vi "Create Output Channels.vi"(8 "error in (no error)":errorcluster, 11 "DAQmx Lockin Digitizer Driver in":refnum<class "DAQmx Lockin Digitizer Driver.lvclass">) -> (0 "error out":errorcluster, 3 "DAQmx Lockin Digitizer Driver out":refnum<class "DAQmx Lockin Digitizer Driver.lvclass">)   [LabVIEW 2021, in "DAQmx Lockin Digitizer Driver.lvclass"]
uses:
  DAQmx Lockin Digitizer Driver.lvclass
  C:/GitHub/NHMFL_Core/Libraries/Instruments/Pulse Driver/Lockin Digitizer Driver/Lockin Digitizer Driver.lvclass
  C:/GitHub/NHMFL_Core/Libraries/NI-DAQ/DAQmx Digitizer/DAQmx Digitizer.lvclass
  C:/GitHub/NHMFL_Core/Libraries/Instruments/Pulse Driver/Pulse Driver.lvclass
  DAQmx Digitizer/DAQmx Digitizer.lvclass/DAQmx Digitizer.ctl
  <vilib>/DAQmx/write.llb/DAQmx Write (Analog 2D DBL NChan NSamp).vi
  DAQmx Digitizer/Read DAQmx Device Name.vi
  <vilib>/DAQmx/create/channels.llb/DAQmx Create Channel (AO-Voltage-Basic).vi
  <vilib>/DAQmx/configure/timing.llb/DAQmx Timing (Sample Clock).vi
  <vilib>/DAQmx/miscellaneous.llb/DAQmx Fill In Error Info.vi
  DAQmx Lockin Digitizer Driver.lvclass/DAQmx Lockin Digitizer Driver.ctl
  <vilib>/Analysis/NI_AALBase.lvlib
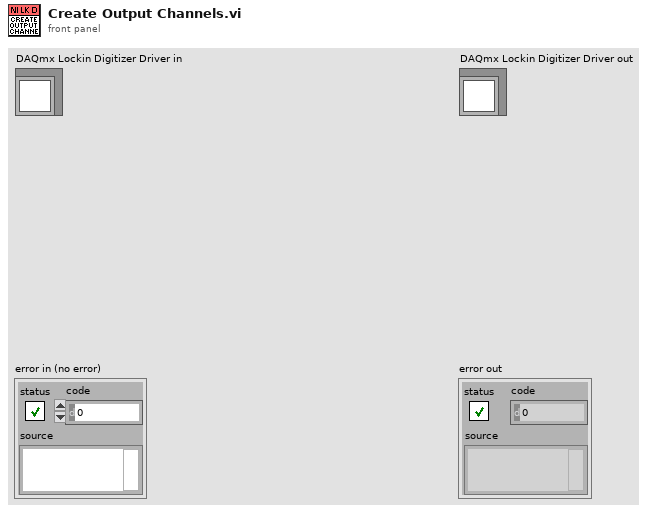
[diagram p1: front panel]
types:
  T1 = typedef "Lockin Digitizer Configuration.ctl" = cluster{"Post-trigger delay":dbl, "Post-trigger duration":dbl, "Rate":dbl, "Ranges":dbl[], "Re-name channels":string[], "Active channels":string, "External\nclock":bool, "Frequencies":dbl[], "Monitor time\nconstant":dbl, "Output \namplitudes":dbl[], "Input\nchannles":string[], "Sync":bool, "Lock-in input channel phases":dbl[]}
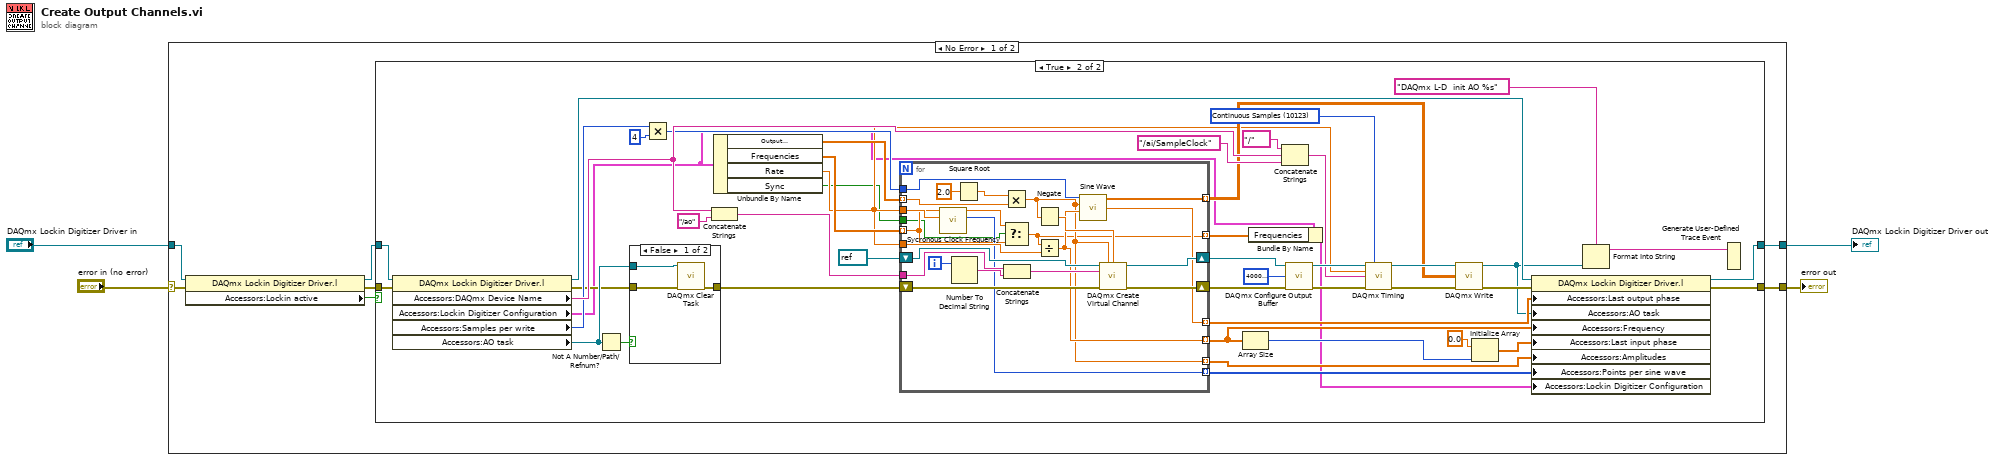
[diagram p0: block diagram]
diagram:
  n1 = case shown="No Error" "error in (no error)" {
    selector: "error in (no error)" -> [w6 w89]
    tunnel: [w9 w89] -> w3
    tunnel: [w10 w88] -> w1
    tunnel: "DAQmx Lockin Digitizer Driver in" -> [w7 w88]
    frame No Error {
      n2 = property class="DAQmx Lockin Digitizer Driver.l"(reference=w7, error in=w6) -> (reference out=w8:refnum<class "DAQmx Lockin Digitizer Driver.lvclass">, error out=w5:errorcluster, "Accessors:Lockin active"=w11:bool)
      n3 = case shown="True" w11 {
        tunnel: w5 -> [w13 w59]
        tunnel: w8 -> [w12 w58]
        tunnel: [w12 w34] -> w10
        tunnel: [w13 w33] -> w9
        frame False {
        }
        frame True {
          w44 = 10123 items=["Finite Samples"=10178, "Continuous Samples"=10123, "Hardware Timed Single Point"=12522] ("sample mode")
          n4 = property class="DAQmx Lockin Digitizer Driver.l"(reference=w58, error in=w59) -> (reference out=w37:refnum<class "DAQmx Lockin Digitizer Driver.lvclass">, error out=w24:errorcluster, "Accessors:DAQmx Device Name"=w46:tag, "Accessors:Lockin Digitizer Configuration"=w16:T1, "Accessors:Samples per write"=w42:i32, "Accessors:AO task"=w25:refnum<k21>)
          n5 = Not A Number/Path/Refnum?(number/path/refnum=w25) -> (NaN/Path/Refnum?=w26:bool)
          n6 = case shown="False" w26 {
            tunnel: w25 -> [w62 _]
            tunnel: w24 -> [w61 w63]
            tunnel: [w60 w63] -> w23
            frame False {
              n7 = call <vilib>:"DAQmx Clear Task.vi"("task in"=w62, "error in"=w61) -> ("error out"=w60:errorcluster)  [unwired: 13 in]
            }
            frame True {
            }
          }
          n8 = Multiply(x=w42, y=4) -> (x*y=w41:i32)
          n9 = Concatenate Strings(w46, "/ao" ("string")) -> (w54:string)
          n10 = Unbundle By Name(w16) -> ("Output \namplitudes"=w55:dbl[], "Frequencies"=w32:dbl[], "Rate"=w19:dbl, "Sync"=w17:bool)
          n11 = for {
            shift-right: [w84] -> w53
            shift-left: w23 -> [w87]
            shift-right: [w85] -> w51
            shift-left: refnum<k21> refnum ("task out") -> [w83]
            tunnel: w32 -> [w66] mode=indexing
            tunnel: w55 -> [w79] mode=indexing
            tunnel: w54 -> [w77]
            tunnel: w41 -> [w75]
            tunnel: w19 -> [w74]
            tunnel: [w73] -> w36 mode=indexing
            tunnel: [w72] -> w38 mode=indexing
            tunnel: [w71] -> w31 mode=indexing
            tunnel: [w70] -> w27 mode=indexing
            tunnel: w19 -> [w69]
            tunnel: [w67] -> w18 mode=indexing
            tunnel: w17 -> [w65]
            tunnel: [w64] -> w15 mode=indexing
            i -> [w78]
            n12 = call "Sycronous Clock Frequency.vi"("Clock"=w69, "Frequency in"=w66) -> ("Points per sine wave"=w67:i32, "Frequency out"=w68:dbl)  [unwired: 8 in]
            n13 = Number To Decimal String(number=w78) -> (decimal integer string=w80:string)  [unwired: 1 in]
            n14 = Square Root(x=2.0) -> (sqrt(x)=w82:dbl)
            n15 = Multiply(x=w82, y=w79) -> (x*y=w70:dbl)
            n16 = Select(t=w68, s=w65, f=w66) -> (s? t:f=w64:dbl)
            n17 = Concatenate Strings(w77, w80) -> (w76:string)
            n18 = Negate(x=w70) -> (-x=w86:dbl)
            n19 = Divide(x=w64, y=w74) -> (x/y=w71:dbl)
            n20 = call <vilib>:"Sine Wave.vi"("samples"=w75, "amplitude"=w70, "frequency"=w71) -> ("sine wave"=w72:dbl[], "phase out"=w73:dbl)  [unwired: 2 in, 1 out]
            n21 = call-poly <vilib>:"DAQmx Create Virtual Channel.vi"("task in"=w83, "maximum value"=w70, "minimum value"=w86, "physical channels"=w76, "error in"=w87) -> ("task out"=w85:refnum<k21>, "error out"=w84:errorcluster)  [unwired: 9 in]
          }
          n22 = Array Size(array=w31) -> (size(s)=w30:i32)
          n23 = Bundle By Name(cluster=w16, "Frequencies"=w15) -> (w14:T1)
          n24 = Concatenate Strings(tag "/" ("string"), w46, "/ai/SampleClock" ("string")) -> (w45:string)
          n25 = call <vilib>:"DAQmx Configure Output Buffer.vi"("task/channels in"=w51, "buffer size (in samples per channel)"=u32 40000000, "error in"=w53) -> ("task out"=w49:refnum<k21>, "error out"=w50:errorcluster)  [unwired: 11 in]
          n26 = call-poly <vilib>:"DAQmx Timing.vi"("task/channels in"=w49, "sample mode"=w44, "rate"=w19, "source"=w45, "error in"=w50) -> ("task out"=w39:refnum<k21>, "error out"=w40:errorcluster)  [unwired: 9 in]
          n27 = call-poly <vilib>:"DAQmx Write.vi"("task/channels in"=w39, "data"=w38, "error in"=w40) -> ("task out"=w20:refnum<k21>, "error out"=w35:errorcluster)  [unwired: 10 in, 1 out]
          n28 = Initialize Array(0.0 ("element"), w30) -> (w28:dbl[])
          n29 = property class="DAQmx Lockin Digitizer Driver.l"(reference=w37, error in=w35, "Accessors:Last output phase"=w36, "Accessors:AO task"=w20, "Accessors:Frequency"=w31, "Accessors:Last input phase"=w28, "Accessors:Amplitudes"=w27, "Accessors:Points per sine wave"=w18, "Accessors:Lockin Digitizer Configuration"=w14) -> (reference out=w34:refnum<class "DAQmx Lockin Digitizer Driver.lvclass">, error out=w33:errorcluster)
          n30 = Format Into String(format string="DAQmx L-D  init AO %s" ("string"), w20) -> (resulting string=w21:string)  [unwired: 2 in, 1 out]
          n31 = Generate User-Defined Trace Event(2:w21) -> ()  [unwired: 1 in]
        }
      }
    }
    frame Error {
    }
  }
  "error out" <- w3
  "DAQmx Lockin Digitizer Driver out" <- w1
